vi "CheckTACommand.vi"(4 "error in (no error)":errorcluster, 5 "Wait before read (0ms)":u32=10, 6 "Axis (1)":i32=1 min=1 max=3, 7 "VISA resource name":refnum<visa-resource-name>) -> (0 "error out":errorcluster, 2 "Returned string":string, 3 "VISA resource name out":refnum<visa-resource-name>)   [LabVIEW 2011]
doc: "Returns the DAC offset value."
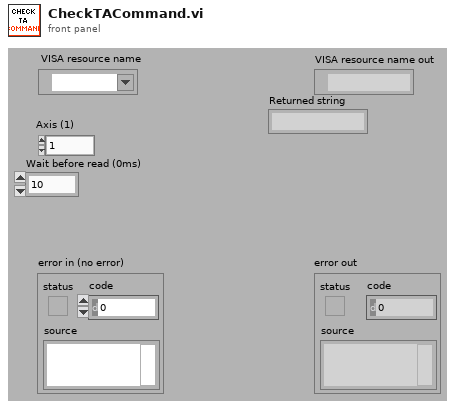
[diagram p1: front panel]
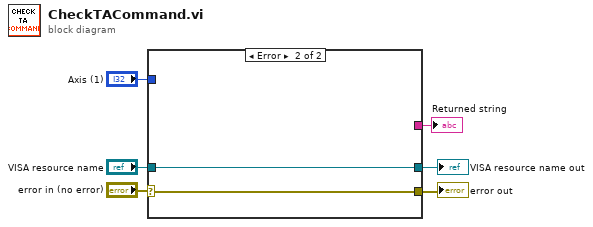
[diagram p0: block diagram]
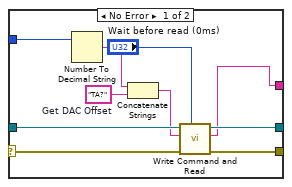
[diagram p2: hidden frame]
diagram:
  n1 = case shown="Error" "error in (no error)" {
    selector: "error in (no error)" -> [w13 w18]
    tunnel: [w15 w18] -> w6
    tunnel: "VISA resource name" -> [w16 w17]
    tunnel: [w14 w17] -> w5
    tunnel: [w7 _] -> w1
    tunnel: "Axis (1)" -> [w10 _]
    frame No Error {
      w12 = "TA?"  # Get DAC Offset
      n2 = Number To Decimal String(number=w10) -> (decimal integer string=w11:string)  [unwired: 1 out]
      n3 = Concatenate Strings(w11, w12) -> (w9:string)
      n4 = call <instrlib>:"Write Command and Read.vi"("Wait before read (0ms)"="Wait before read (0ms)", "error in (no error)"=w13, "Command"=w9, "VISA resource name"=w16) -> ("error out"=w15:errorcluster, "Returned string"=w7:string, "VISA resource name out"=w14:refnum<visa-resource-name>)  [unwired: 1 in, 2 out]
    }
    frame Error {
    }
  }
  "error out" <- w6
  "VISA resource name out" <- w5
  "Returned string" <- w1
